vi "Read 1Port 1Sampe 1D Boolean.vi"(8 "error in (no error)":errorcluster, 10 "Port (Bank)":T1=1 items=["DIO1...8"=1, "DIO9...16"=2, "DIO17...24"=3, "DIO25...32"=4], 11 "MicroDAQ.lvlib:Digital Input.lvclass":refnum<class "Digital Input.lvclass">) -> (0 "error out":errorcluster, 2 "data":bool[](array[boolean]), 3 "MicroDAQ.lvlib:Digital Input.lvclass out":refnum<class "Digital Input.lvclass">)   [LabVIEW 2009, in "MicroDAQ.lvlib" / "Digital Input.lvclass"]
doc: "Reads a U8 register value from a digital input channel composed of a single port."
uses:
  <instrlib>/MicroDAQ/Channel/Digital Input/Digital Input.lvclass
  <instrlib>/MicroDAQ/Tools/Digital IO channels.ctl
  <instrlib>/MicroDAQ/Mlink library wraper/mlink.lvlib
  <instrlib>/MicroDAQ/Channel/Channel.lvclass
  <instrlib>/MicroDAQ/MicroDAQ.lvlib
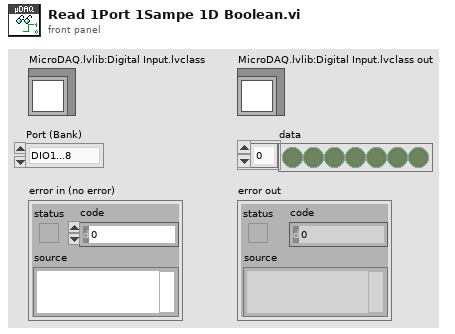
[diagram p1: front panel]
types:
  T1 = typedef "MicroDAQ.lvlib/Digital IO channels.ctl" = u8
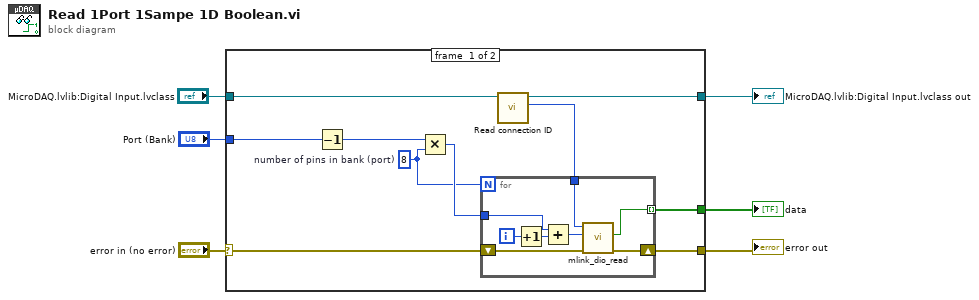
[diagram p0: block diagram]
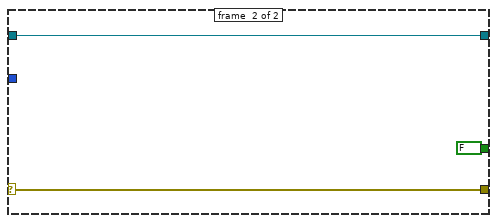
[diagram p2: hidden frame]
diagram:
  n1 = case shown="No Error" "error in (no error)" {
    selector: "error in (no error)" -> [w11 w25]
    tunnel: [w16 w25] -> w5
    tunnel: "MicroDAQ.lvlib:Digital Input.lvclass" -> [w12 w26]
    tunnel: [w15 w26] -> w3
    tunnel: [w13 _] -> w1
    tunnel: "Port (Bank)" -> [w10 _]
    frame #0 {
      w8 = 8  # number of pins in bank (port)
      n2 = Decrement(x=w10) -> (x-1=w7:T1)
      n3 = Multiply(x=w7, y=w8) -> (x*y=w9:i32)
      n4 = call <instrlib>:"Read connection ID.vi"("Task in"=w12) -> ("connection ID"=w14:i32, "Task out"=w15:refnum<class "Digital Input.lvclass">)  [unwired: 9 in]
      n5 = for {
        N: w8 -> [_]
        tunnel: w14 -> [w23]
        tunnel: [w22] -> w13 mode=indexing
        shift-right: [w24] -> w16
        shift-left: w11 -> [w21]
        tunnel: w9 -> [w18]
        i -> [w19]
        n6 = Increment(x=w19) -> (x+1=w17:i32)
        n7 = Add(x=w18, y=w17) -> (x+y=w20:i32)
        n8 = call <instrlib>:"mlink_dio_read.vi"("error in (no error)"=w21, "pin"=w20, "connection ID"=w23) -> ("error out"=w24:errorcluster, "state"=w22:bool)  [unwired: 6 in, 1 out]
      }
    }
    frame #1 {
      (unwired) FALSE ("state")
    }
  }
  "error out" <- w5
  "MicroDAQ.lvlib:Digital Input.lvclass out" <- w3
  "data" <- w1
